vi "get Ship Textures Hotspots.vi"(11 "Ship in":refnum<class "Ship.lvclass">) -> (3 "Ship Hotspots":refnum<class "Vector 2D.lvclass">[](array[class]))   [LabVIEW 2021, in "Ship.lvclass"]
uses:
  Ship.lvclass
  Ship.lvclass/Ship.ctl
  Vector 2D/Vector 2D.lvclass
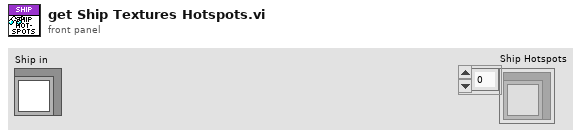
[diagram p1: front panel]
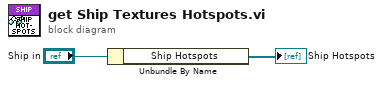
[diagram p0: block diagram]
diagram:
  n1 = Unbundle By Name("Ship in") -> ("Ship Hotspots"=→"Ship Hotspots":refnum<class "Vector 2D.lvclass">[])
